vi "interp_4d.vi"(8 "Input x":sgl[](array[numeric]), 10 "Set LUT":bool, 11 "LUT":T1) -> (2 "Output f(x)":sgl[](array[numeric]) format="%#.2f")   [LabVIEW 2013]
uses:
  lut4d.ctl
panel:
  # "To avoid copying of LUT, it is only passed once at system initialization (when \"Set LUT\" is true.)"
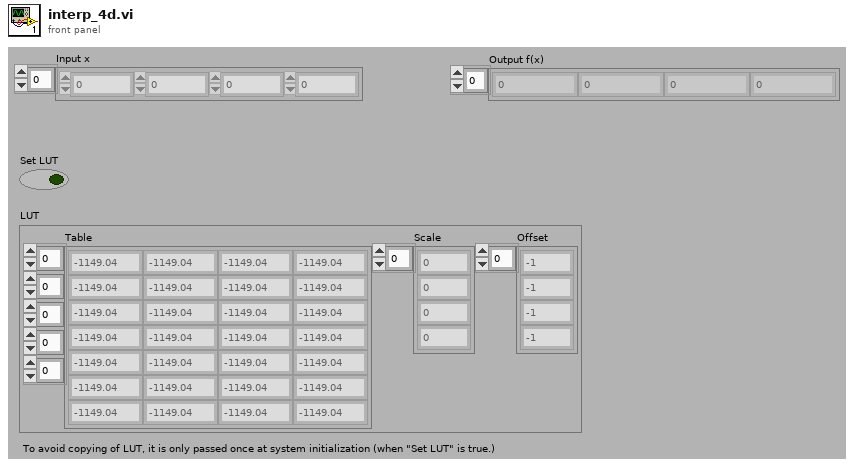
[diagram p1: front panel]
types:
  T1 = typedef "lut4d.ctl" = cluster{"Table":sgl[][][][][], "Scale":sgl[], "Offset":sgl[]}
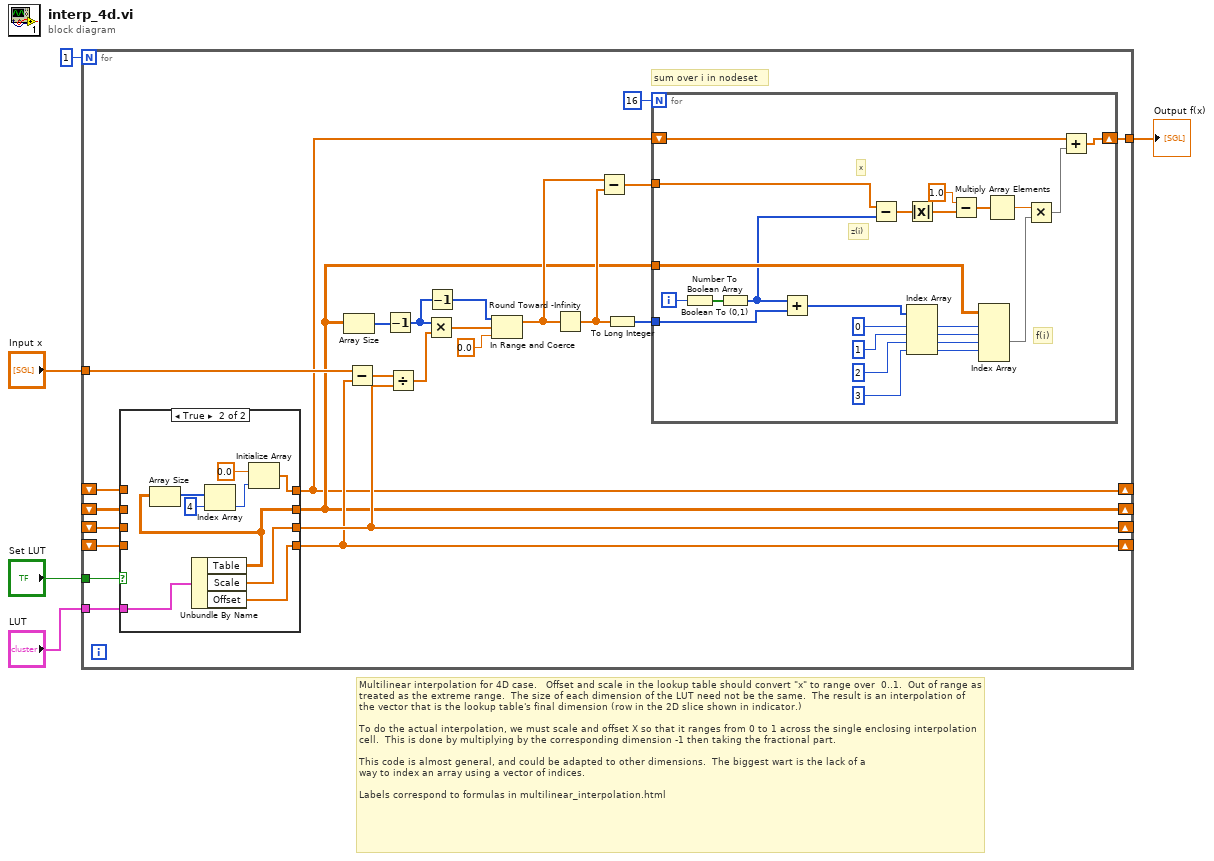
[diagram p0: block diagram]
diagram:
  # "Multilinear interpolation for 4D case.   Offset and scale in the lookup table should convert \"x\" to range over  0..1.  Out of range as treated as the extreme range.  The size of each dimension of the LUT need not be the same.  The result is an interpolation of the vector that is the lookup table's final dimension (row in the 2D slice shown in indicator.)\n\nTo do the actual interpolation, we must scale and offset X so that it ranges from 0 to 1 across the single enclosing interpolation cell.  This is done by multiplying by the corresponding dimension -1 then taking the fractional part.\n\nThis code is almost general, and could be adapted to other dimensions.  The biggest wart is the lack of a \nway to index an array using a vector of indices.\n\nLabels correspond to formulas in multilinear_interpolation.html"
  n1 = for {
    N: 1 -> [_]
    tunnel: "Input x" -> [w23]
    shift-right: [w8] -> _
    shift-left: _ -> [w10]
    shift-right: [w16] -> _
    shift-left: _ -> [w13]
    shift-right: [w15] -> _
    shift-left: _ -> [w12]
    tunnel: "Set LUT" -> [w14]
    tunnel: [w11] -> w2
    tunnel: "LUT" -> [w9]
    shift-right: [w6] -> _
    shift-left: _ -> [w7]
    # "sum over i in nodeset"
    n2 = case shown="True" w14 {
      tunnel: [w33 w39] -> w8
      tunnel: [w32 w42] -> w16
      tunnel: [w31 w41] -> w15
      tunnel: w10 -> [w33 _]
      tunnel: w13 -> [w32 _]
      tunnel: w12 -> [w31 _]
      tunnel: w9 -> [_ w40]
      tunnel: [w30 w34] -> w6
      tunnel: w7 -> [w30 _]
      frame False {
      }
      frame True {
        n3 = Unbundle By Name(w40) -> ("Table"=w39:sgl[][][][][], "Scale"=w42:sgl[], "Offset"=w41:sgl[])
        n4 = Array Size(array=w39) -> (size(s)=w38:i32[])
        n5 = Index Array(array=w38, index=4) -> (element=w36:i32)
        n6 = Initialize Array(sgl 0.0, w36) -> (w34:sgl[])
      }
    }
    n7 = Array Size(array=w8) -> (size(s)=w26:i32[])
    n8 = Subtract(x=w23, y=w15) -> (x-y=w24:sgl[])
    n9 = Decrement(x=w26) -> (x-1=w18:i32[])
    n10 = Divide(x=w24, y=w16) -> (x/y=w21:sgl[])
    n11 = Multiply(x=w18, y=w21) -> (x*y=w19:sgl[])
    n12 = Decrement(x=w18) -> (x-1=w17:i32[])
    n13 = In Range and Coerce(upper limit=w17, x=w19, lower limit=sgl 0.0) -> (coerced(x)=w20:sgl[])  [unwired: 1 out]
    n14 = Round Toward -Infinity(1:w20) -> (0:w27:sgl[])
    n15 = Subtract(x=w20, y=w27) -> (x-y=w28:sgl[])
    n16 = To Long Integer(number=w27) -> (32bit integer=w29:i32[])
    n17 = for {
      N: 16 -> [_]
      tunnel: w29 -> [w46]
      tunnel: w8 -> [w62]
      shift-right: [w50] -> w11
      shift-left: w6 -> [w51]
      tunnel: w28 -> [w45]
      i -> [w49]
      # "x"
      # "z(i)"
      # "f(i)"
      n18 = Number To Boolean Array(number=w49) -> (Boolean array=w66:bool[])
      n19 = Boolean To (0,1)(Boolean=w66) -> (0, 1=w48:i16[])
      n20 = Add(x=w48, y=w46) -> (x+y=w47:i32[])
      n21 = Subtract(x=w45, y=w48) -> (x-y=w58:sgl[])
      n22 = Absolute Value(x=w58) -> (abs(x)=w57:sgl[])
      n23 = Index Array(array=w47, index #1=0 ("index"), index #2=1 ("index"), index #3=2 ("index"), index #4=3 ("index")) -> (element #1=w61:i32, element #2=w60:i32, element #3=w59:i32, element #4=w43:i32)
      n24 = Subtract(x=sgl 1.0, y=w57) -> (x-y=w55:sgl[])
      n25 = Index Array(array=w62, index (dim 0)=w61, index (dim 1)=w60, index (dim 2)=w59, index (dim 3)=w43) -> (element=w53:sgl[])  [unwired: 1 in]
      n26 = Multiply Array Elements(1:w55) -> (0:w54:sgl)
      n27 = Multiply(x=w54, y=w53) -> (x*y=w52:sgl[])
      n28 = Add(x=w51, y=w52) -> (x+y=w50:sgl[])
    }
  }
  "Output f(x)" <- w2
